vi "Find Intensity Peaks V2.vi"(0 "Data In":dbl[](array[numeric]), 1 "Gaussian Fit Method":T2 items=["Least Square", "Least Absolute Residual", "Bisquare"], 2 "Intensity Threshold":i32, 3 "error in (no error)":errorcluster, 4 "Fit Range":u32[](array[numeric])) -> (5 "Peak Find Comparison":cluster{"Locations":dbl[], "Amplitudes":dbl[]}[](array[cluster]), 6 "Gaussian Fit Results":T1, 7 "error out":errorcluster)   [LabVIEW 2012]
uses:
  <vilib>/Analysis/6fits.llb/Curve Fitting Criteria.ctl
  <userlib>/_OpenG.lib/array/array.llb/Slice 1D Array (DBL)__ogtk.vi
  <vilib>/Analysis/NI_AAL_SigProc.lvlib
  <vilib>/Analysis/NI_AALPro.lvlib
panel:
  in  "Peak Detector Width":i32=3 min=3
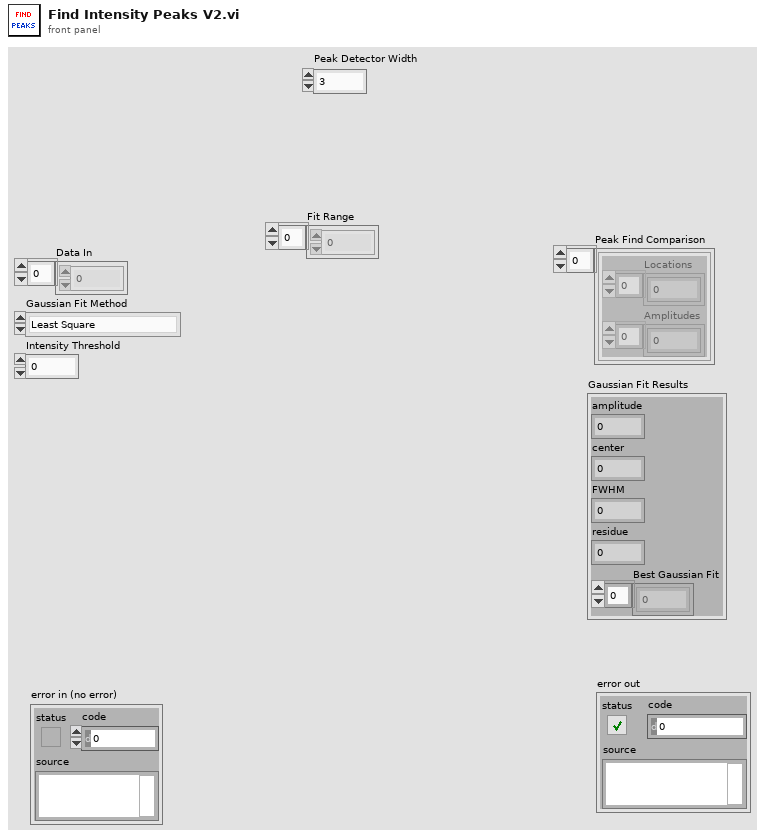
[diagram p1: front panel]
types:
  T1 = cluster{"amplitude":dbl, "center":dbl, "FWHM":dbl, "residue":dbl, "Best Gaussian Fit":dbl[]}
  T2 = typedef "NI_AALPro.lvlib/Curve Fitting Criteria.ctl" = u16
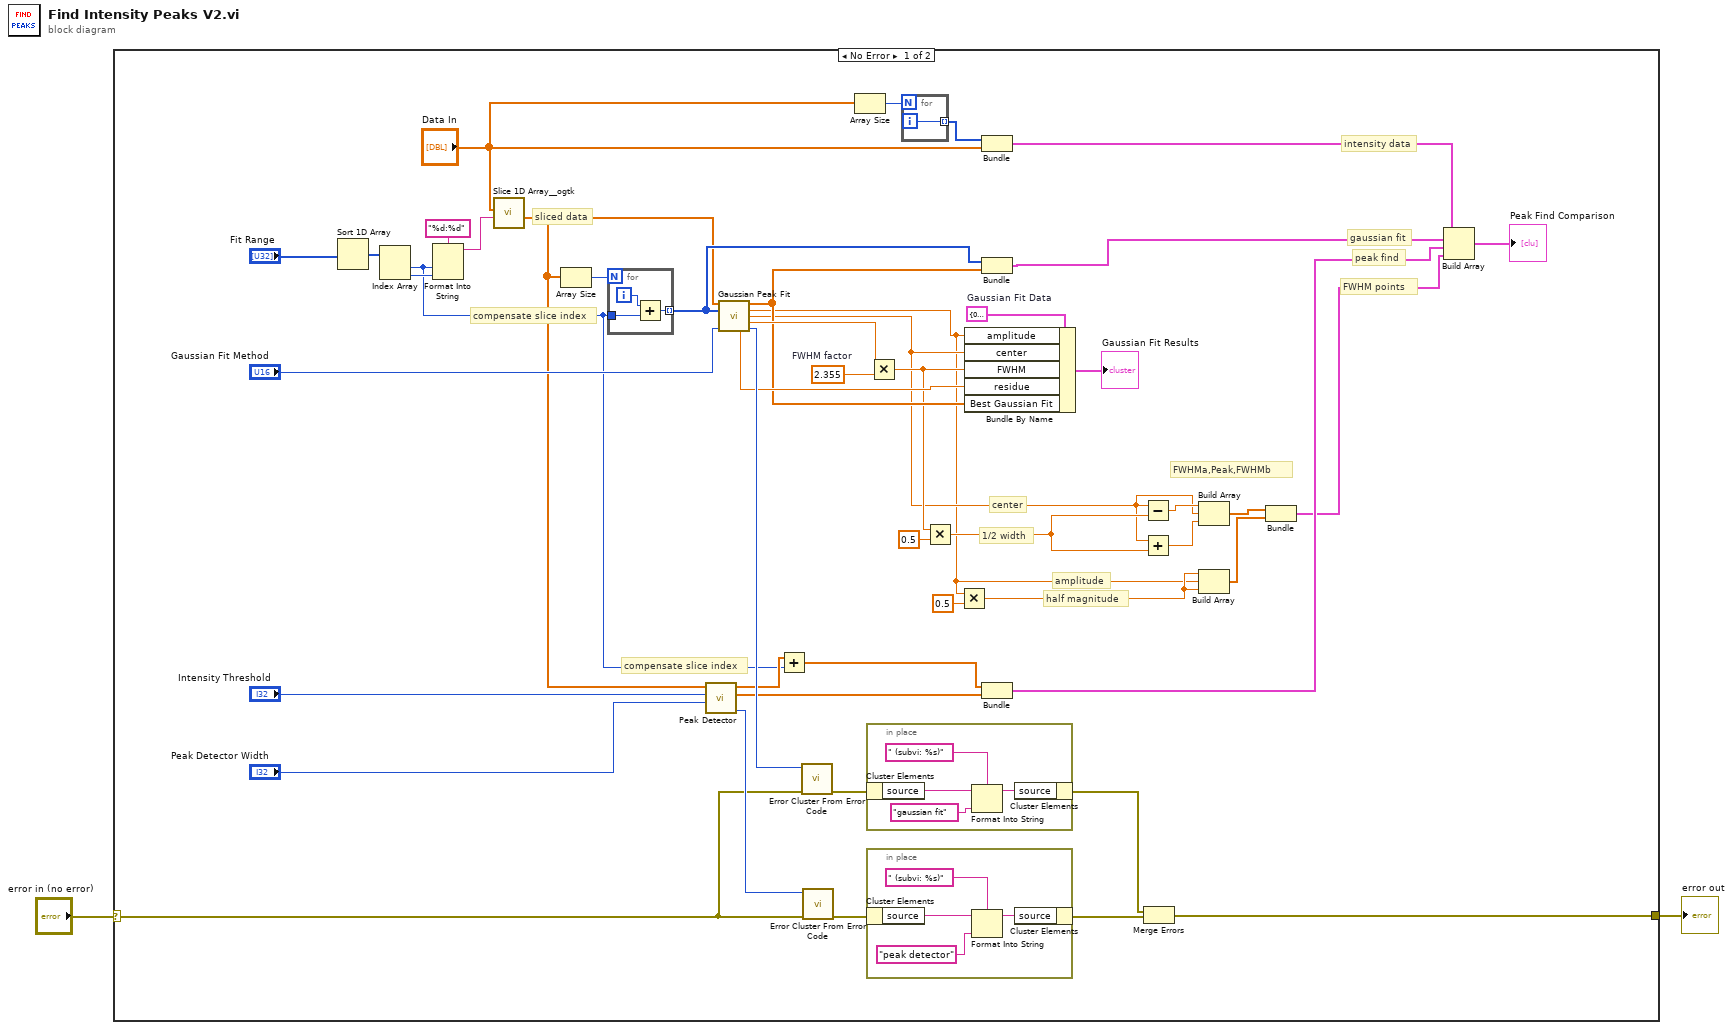
[diagram p0: block diagram]
diagram:
  n1 = case shown="No Error" "error in (no error)" {
    selector: "error in (no error)" -> [w3 w63]
    tunnel: [w4 w63] -> w2
    frame No Error {
      w37 = T1 {"amplitude"=0.0, "center"=0.0, "FWHM"=0.0, "residue"=0.0, "Best Gaussian Fit"=[]}  # Gaussian Fit Data
      w39 = 2.355  # FWHM factor
      # "compensate slice index"
      # "compensate slice index"
      # "FWHM points"
      # "sliced data"
      # "amplitude"
      # "1/2 width"
      # "FWHMa,Peak,FWHMb"
      # "half magnitude"
      # "center"
      # "peak find"
      # "gaussian fit"
      # "intensity data"
      n2 = Sort 1D Array(array="Fit Range") -> (sorted array=w21:u32[])
      n3 = Index Array(array=w21) -> (element #1=w10:u32, element #2=w22:u32)  [unwired: 2 in]
      n4 = Format Into String(format string="%d:%d", w10, w22) -> (resulting string=w19:string)  [unwired: 2 in, 1 out]
      n5 = call-poly <userlib>:"Slice 1D Array__ogtk.vi"("slice"=w19, "array"="Data In") -> ("subarray (array[i:j])"=w15:dbl[])  [unwired: 5 in]
      n6 = Array Size(array=w15) -> (size(s)=w42:i32)
      n7 = for {
        N: w42 -> [_]
        tunnel: [w61] -> w45 mode=indexing
        tunnel: w10 -> [w60]
        i -> [w62]
        n8 = Add(x=w62, y=w60) -> (x+y=w61:u32)
      }
      n9 = call <vilib>:"Peak Detector.vi"("width"="Peak Detector Width", "threshold"="Intensity Threshold", "X"=w15) -> ("error"=w40:i32, "Amplitudes"=w48:dbl[], "Locations"=w11:dbl[])  [unwired: 4 in, 2 out]
      n10 = call <vilib>:"Gaussian Peak Fit.vi"("Y"=w15, "X"=w45, "method"="Gaussian Fit Method") -> ("Best Gaussian Fit"=w35:dbl[], "amplitude"=w23:dbl, "center"=w26:dbl, "standard deviation"=w38:dbl, "residue"=w36:dbl, "error"=w50:i32)  [unwired: 6 in, 1 out]
      n11 = Add(x=w11, y=w10) -> (x+y=w9:dbl[])
      n12 = call <vilib>:"Error Cluster From Error Code.vi"("error in (no error)"=w3, "error code (0)"=w50) -> ("error out"=w8:errorcluster)  [unwired: 7 in]
      n13 = call <vilib>:"Error Cluster From Error Code.vi"("error in (no error)"=w3, "error code (0)"=w40) -> ("error out"=w7:errorcluster)  [unwired: 7 in]
      n14 = Array Size(array="Data In") -> (size(s)=w17:i32)
      n15 = in-place "In Place Element Structure" {
        n16 = in-place-cluster #1(w8) -> ("source"=w56:string)
        n17 = Format Into String(format string=" (subvi: %s)" ("initial string"), initial string=w56, "gaussian fit" ("input 1")) -> (resulting string=w58:string)  [unwired: 1 in, 1 out]
        n18 = in-place-cluster #1("source"=w58) -> (w5:errorcluster)
      }
      n19 = in-place "In Place Element Structure" {
        n20 = in-place-cluster #2(w7) -> ("source"=w52:string)
        n21 = Format Into String(format string=" (subvi: %s)" ("initial string"), initial string=w52, "peak detector" ("input 1")) -> (resulting string=w54:string)  [unwired: 1 in, 1 out]
        n22 = in-place-cluster #2("source"=w54) -> (w6:errorcluster)
      }
      n23 = Multiply(x=w38, y=w39) -> (x*y=w30:dbl)
      n24 = for {
        N: w17 -> [_]
        tunnel: [w59] -> w16 mode=indexing
        i -> [w59]
      }
      n25 = Multiply(x=w30, y=0.5) -> (x*y=w28:dbl)
      n26 = Multiply(x=w23, y=0.5) -> (x*y=w24:dbl)
      n27 = Bundle By Name(cluster=w37, "amplitude"=w23, "center"=w26, "FWHM"=w30, "residue"=w36, "Best Gaussian Fit"=w35) -> (→"Gaussian Fit Results":T1)
      n28 = Bundle(w16, "Data In"="Data In") -> (w44:cluster{i32[], "Data In":dbl[]})  [unwired: 1 in]
      n29 = Bundle(w45, "Best Gaussian Fit"=w35) -> (w46:cluster{u32[], "Best Gaussian Fit":dbl[]})  [unwired: 1 in]
      n30 = Bundle(w9, "Amplitudes"=w48) -> (w13:cluster{dbl[], "Amplitudes":dbl[]})  [unwired: 1 in]
      n31 = Subtract(x=w26, y=w28) -> (x-y=w32:dbl)
      n32 = Add(x=w26, y=w28) -> (x+y=w27:dbl)
      n33 = Merge Errors(w5, w6) -> (w4:errorcluster)
      n34 = Build Array(w32, w26, w27) -> (w33:dbl[])
      n35 = Build Array(w24, w23, w24) -> (w31:dbl[])
      n36 = Bundle(w33, w31) -> (w12:cluster{dbl[], dbl[]})  [unwired: 1 in]
      n37 = Build Array(w44, w46, w13, w12) -> (→"Peak Find Comparison":cluster{dbl[], "Amplitudes":dbl[]}[])
    }
    frame Error {
    }
  }
  "error out" <- w2
